vi "Version.vi"(7 "LabVIEW Web Service Request":refnum<class "Web Request.lvclass">) -> ()   [LabVIEW 2016]
uses:
  <vilib>/wsapi/Web Request.lvclass
  C:/Program Files (x86)/National Instruments/LabVIEW 2016/vi.lib/wsapi/Web Service.lvclass
  <vilib>/wsapi/Web Service.lvclass
  Libraries/WSsupport/WSsupport.lvlib
  Libraries/ServerErrors/ServerErrors.lvlib
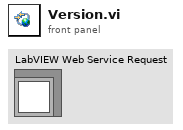
[diagram p1: front panel]
types:
  T1 = typedef "ServerErrors.lvlib/Error Message--cluster.ctl" = cluster{"HTTP Code":i32, "JSON Response":cluster{"error":string, "reason":string}}
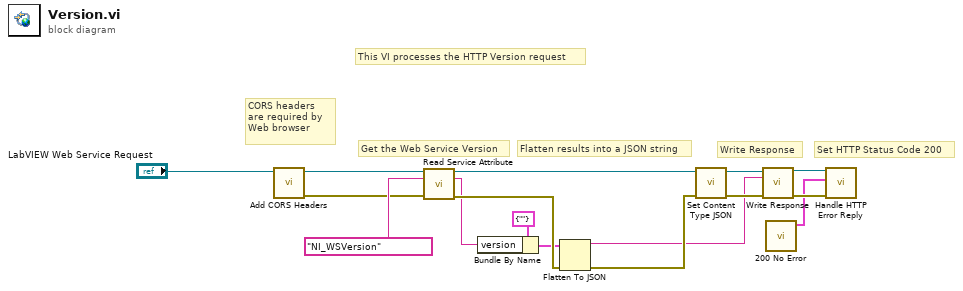
[diagram p0: block diagram]
diagram:
  # "CORS headers are required by Web browser"
  # "Set HTTP Status Code 200"
  # "Write Response"
  # "Flatten results into a JSON string"
  # "Get the Web Service Version"
  # "This VI processes the HTTP Version request"
  n1 = call "Add CORS Headers.vi"("LabVIEW Web Service Request"="LabVIEW Web Service Request") -> ("error out"=w1:errorcluster, "LabVIEW Web Service Request out"=w2:refnum<class "Web Request.lvclass">)  [unwired: 9 in]
  n2 = call <vilib>:"Read Service Attribute.vi"("LabVIEW Web Service"=w2, "attribute name"="NI_WSVersion", "error in (no error)"=w1) -> ("LabVIEW Web Service out"=w14:refnum<class "Web Request.lvclass">, "value"=w10:string, "error out"=w13:errorcluster)  [unwired: 10 in]
  n3 = Bundle By Name(cluster=cluster{"version":string} {"version"=""}, "version"=w10) -> (w9:cluster{"version":string})
  n4 = Flatten To JSON(anything=w9, error in (no error)=w13) -> (JSON string=w6:string, 11:w12:errorcluster)  [unwired: 1 in]
  n5 = call "Set Content Type JSON.vi"("error in (no error)"=w12, "LabVIEW Web Service Request"=w14) -> ("error out"=w7:errorcluster, "LabVIEW Web Service Request out"=w8:refnum<class "Web Request.lvclass">)  [unwired: 8 in]
  n6 = call <vilib>:"Write Response.vi"("LabVIEW Web Service Request"=w8, "response string"=w6, "error in (no error)"=w7) -> ("LabVIEW Web Service Request out"=w5:refnum<class "Web Request.lvclass">, "error out"=w4:errorcluster)  [unwired: 11 in]
  n7 = call "200 No Error.vi"() -> ("no error"=w3:T1)  [unwired: 11 in]
  n8 = call "Handle HTTP Error Reply.vi"("error in (no error)"=w4, "HTTP Status Code"=w3, "Web Request in"=w5) -> ()  [unwired: 8 in, 1 out]
